vi "Exemple_Metrics_Mean_Gamma_Deviance.vi"() -> ()   [LabVIEW 2020]
uses:
  Objet/3 - Model selection and evaluation/3.3 - Metrics and scoring/mean_gamma_deviance/Mean_Gamma_Deviance.vi
panel:
  out "error out":errorcluster caption="sortie d'erreur"
  out "Score":string
  in  "error in (no error)":errorcluster caption="entrée d'erreur (pas d'erreur)"
  in  "mean_gamma_deviance":cluster{"sample_weight":dbl[]}
  in  "y_pred":string[][](array[string])=[["0,5"], ["0,5"], ["2"], ["2"]]
  in  "y_true":string[][](array[string])=[["2"], ["0,5"], ["1"], ["4"]]
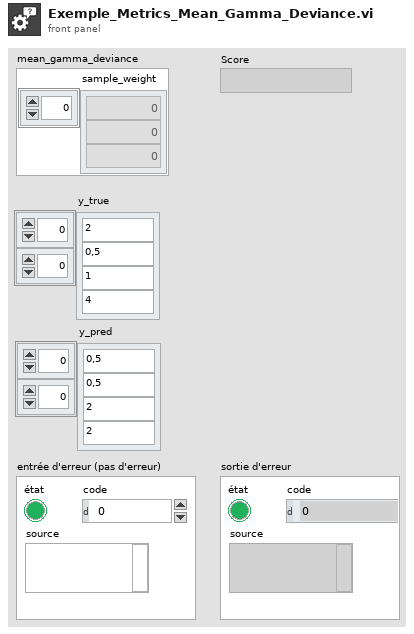
[diagram p1: front panel]
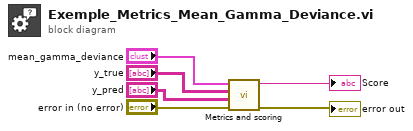
[diagram p0: block diagram]
diagram:
  n1 = call-poly "Metrics and scoring.vi"("error in (no error)"="error in (no error)", "y_pred"="y_pred", "y_true"="y_true", "mean_gamma_deviance"="mean_gamma_deviance") -> ("error out"=→"error out":errorcluster, "Score"=→"Score":string)  [unwired: 6 in]
